vi "Read Allow Transparent.vi"(8 "error in (no error)":errorcluster, 11 "ColorBox.lvclass in":refnum<class "ColorBox.lvclass">) -> (0 "error out":errorcluster, 2 "AllowTransparent":bool, 3 "ColorBox.lvclass out":refnum<class "ColorBox.lvclass">)   [LabVIEW 2015, in "ColorBox.lvclass"]
uses:
  ColorBox.lvclass
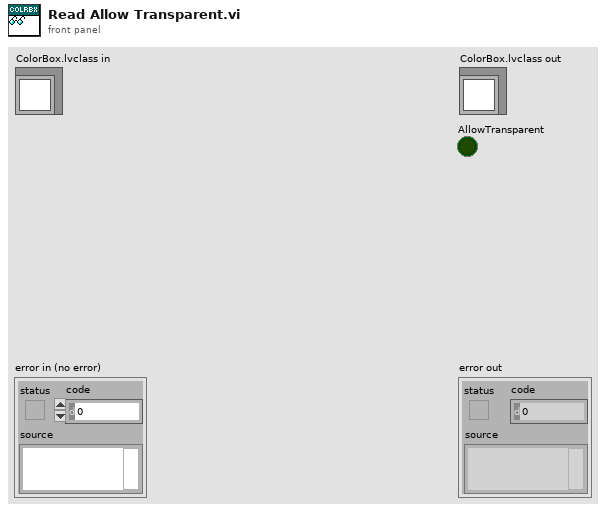
[diagram p1: front panel]
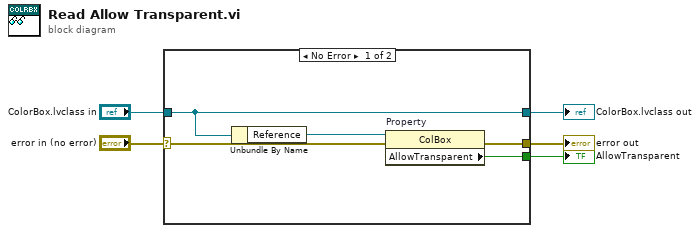
[diagram p0: block diagram]
diagram:
  n1 = case shown="No Error" "error in (no error)" {
    selector: "error in (no error)" -> [w6 w12]
    tunnel: [w9 w12] -> w4
    tunnel: [w8 w11] -> w2
    tunnel: "ColorBox.lvclass in" -> [w8 w11]
    tunnel: [w10 _] -> w1
    frame No Error {
      n2 = Unbundle By Name(w8) -> ("Reference"=w7:refnum<vi>)
      n3 = property on="Property" class="ColBox"(reference=w7, error in=w6) -> (error out=w9:errorcluster, "AllowTransparent"=w10:bool)  [unwired: 1 out]
    }
    frame Error {
    }
  }
  "error out" <- w4
  "ColorBox.lvclass out" <- w2
  "AllowTransparent" <- w1
